vi "graph_data_acquisition_and_display.vi"(1 "input cluster":T2) -> (0 "output cluster":T1)   [LabVIEW 2015]
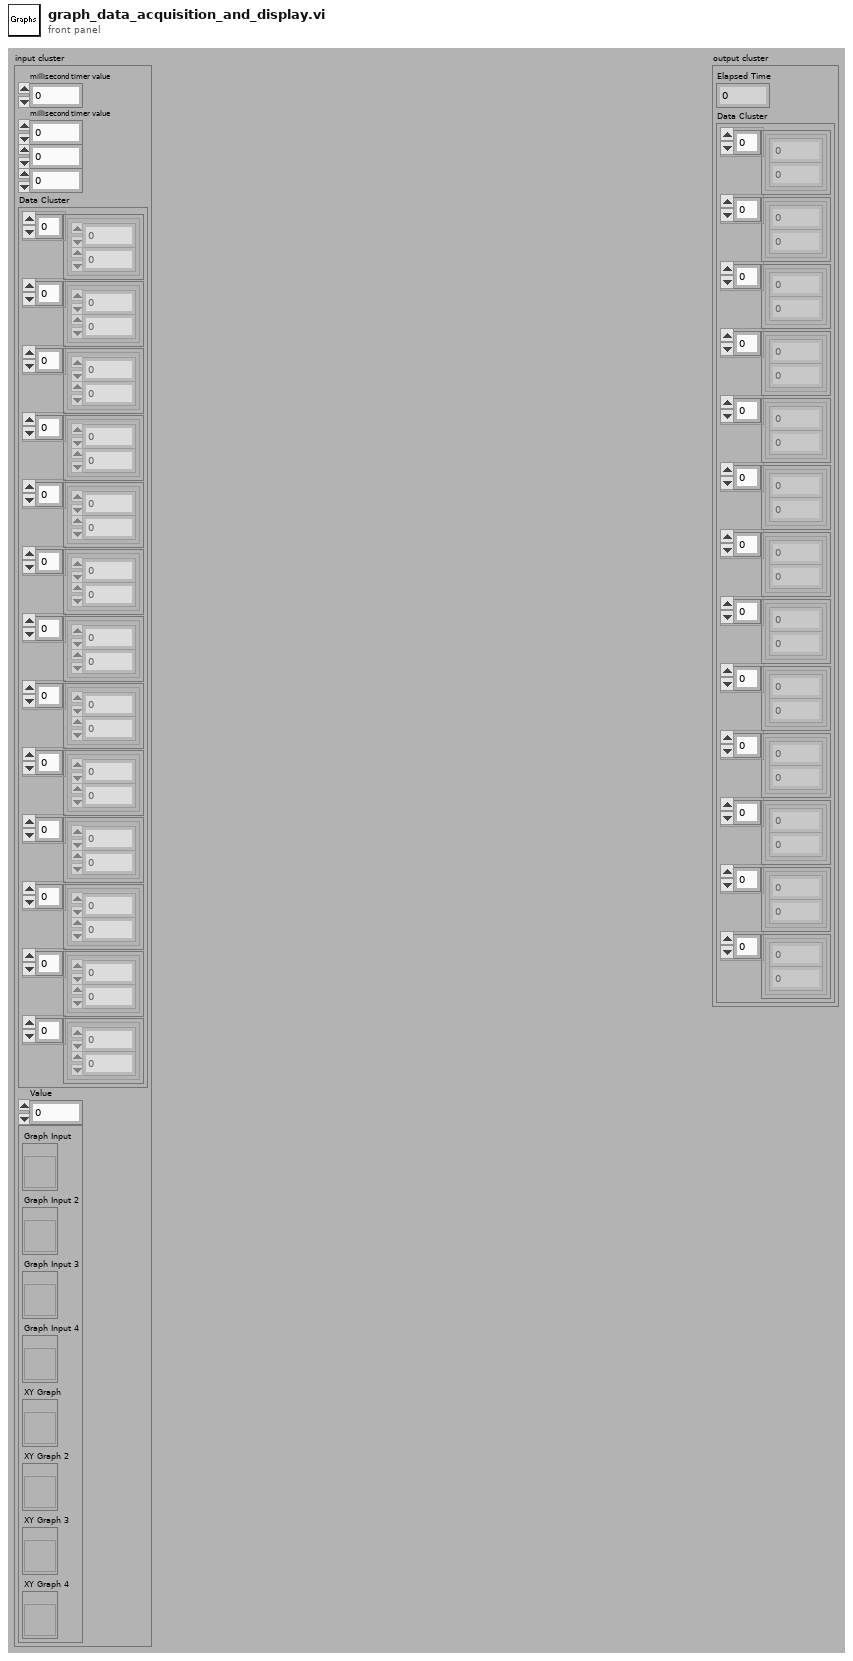
[diagram p1: front panel]
types:
  T1 = cluster{"Elapsed Time":i32, "Data Cluster":cluster{cluster{sgl, sgl}[], cluster{sgl, sgl}[], cluster{sgl, sgl}[], cluster{sgl, sgl}[], cluster{sgl, sgl}[], cluster{sgl, sgl}[], cluster{sgl, sgl}[], cluster{sgl, sgl}[], cluster{sgl, sgl}[], cluster{sgl, sgl}[], cluster{sgl, sgl}[], cluster{sgl, sgl}[], cluster{sgl, sgl}[]}}
  T2 = cluster{"millisecond timer value":u32, "millisecond timer value":u32, i32, sgl, "Data Cluster":cluster{cluster{sgl, sgl}[], cluster{sgl, sgl}[], cluster{sgl, sgl}[], cluster{sgl, sgl}[], cluster{sgl, sgl}[], cluster{sgl, sgl}[], cluster{sgl, sgl}[], cluster{sgl, sgl}[], cluster{sgl, sgl}[], cluster{sgl, sgl}[], cluster{sgl, sgl}[], cluster{sgl, sgl}[], cluster{sgl, sgl}[]}, "Value":i32, cluster{"Graph Input":refnum<vi>, "Graph Input 2":refnum<vi>, "Graph Input 3":refnum<vi>, "Graph Input 4":refnum<vi>, "XY Graph":refnum<vi>, "XY Graph 2":refnum<vi>, "XY Graph 3":refnum<vi>, "XY Graph 4":refnum<vi>}}
  T3 = cluster{cluster{sgl, sgl}[], cluster{sgl, sgl}[], cluster{sgl, sgl}[], cluster{sgl, sgl}[], cluster{sgl, sgl}[], cluster{sgl, sgl}[], cluster{sgl, sgl}[], cluster{sgl, sgl}[], cluster{sgl, sgl}[], cluster{sgl, sgl}[], cluster{sgl, sgl}[], cluster{sgl, sgl}[], cluster{sgl, sgl}[]}
  T4 = cluster{"Graph Input":refnum<vi>, "Graph Input 2":refnum<vi>, "Graph Input 3":refnum<vi>, "Graph Input 4":refnum<vi>, "XY Graph":refnum<vi>, "XY Graph 2":refnum<vi>, "XY Graph 3":refnum<vi>, "XY Graph 4":refnum<vi>}
  T5 = cluster{"Elapsed Time":i32, "output cluster":cluster{cluster{sgl, sgl}[], cluster{sgl, sgl}[], cluster{sgl, sgl}[], cluster{sgl, sgl}[], cluster{sgl, sgl}[], cluster{sgl, sgl}[], cluster{sgl, sgl}[], cluster{sgl, sgl}[], cluster{sgl, sgl}[], cluster{sgl, sgl}[], cluster{sgl, sgl}[], cluster{sgl, sgl}[], cluster{sgl, sgl}[]}}
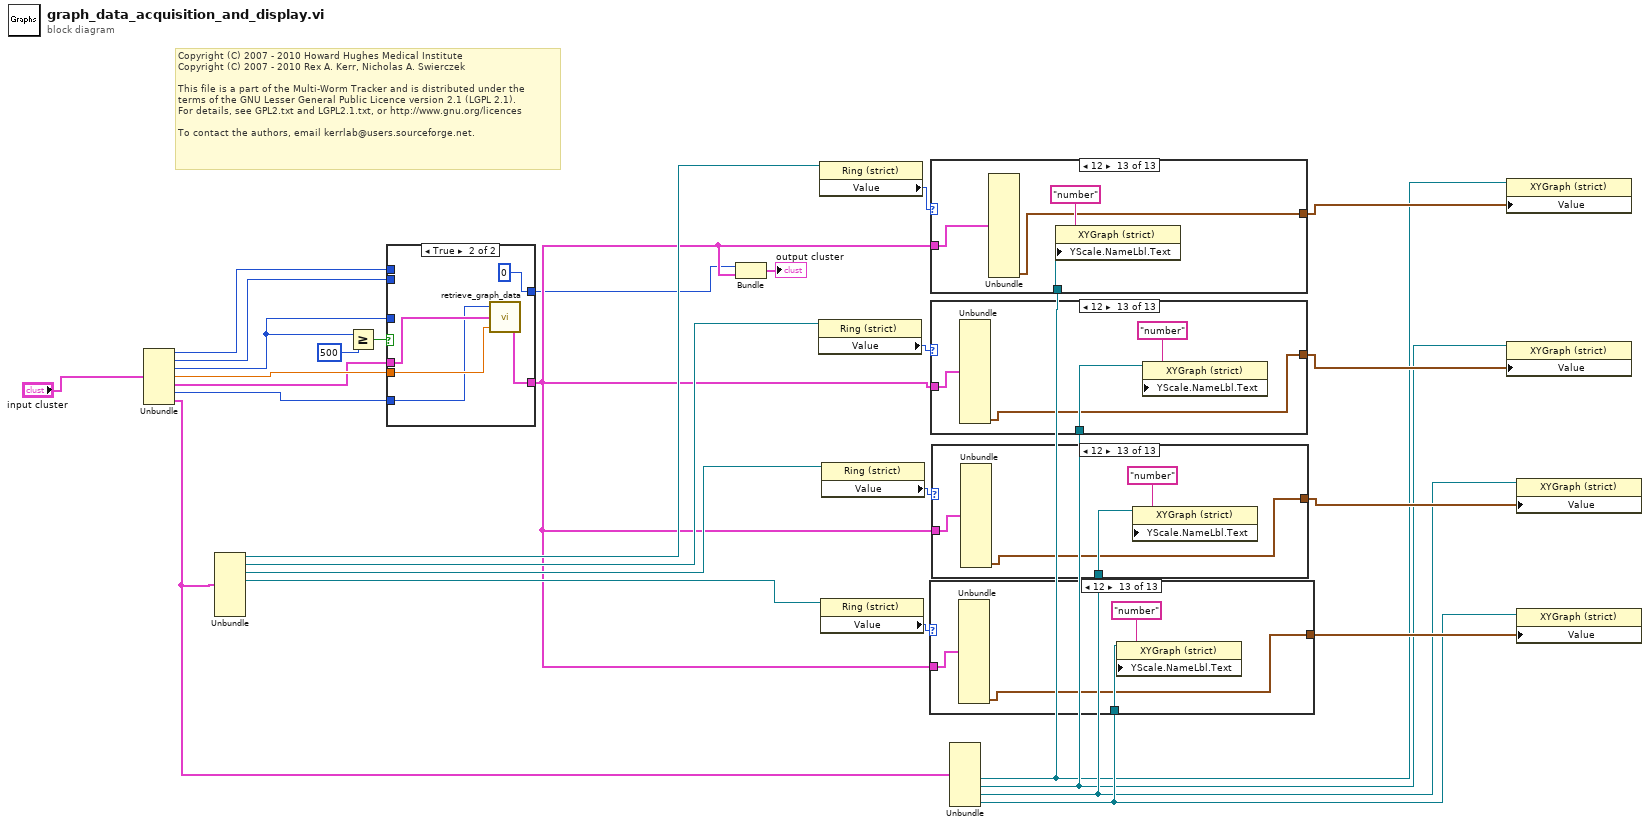
[diagram p0: block diagram]
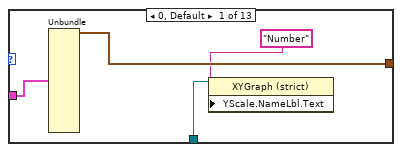
[diagram p2: hidden frame]
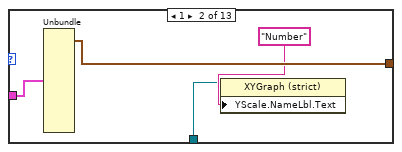
[diagram p3: hidden frame]
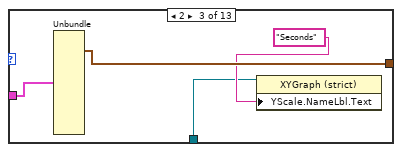
[diagram p4: hidden frame]
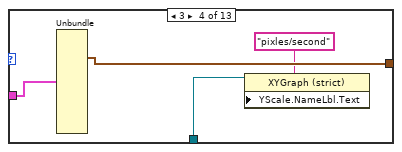
[diagram p5: hidden frame]
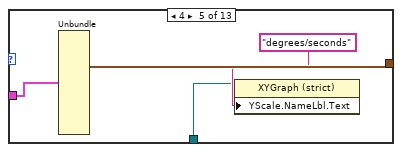
[diagram p6: hidden frame]
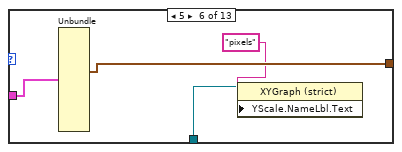
[diagram p7: hidden frame]
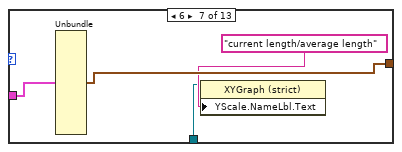
[diagram p8: hidden frame]
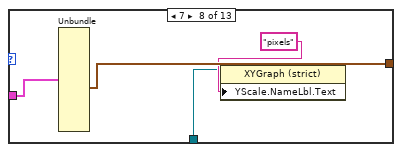
[diagram p9: hidden frame]
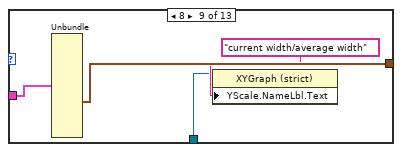
[diagram p10: hidden frame]
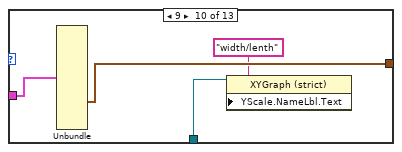
[diagram p11: hidden frame]
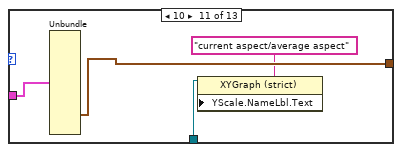
[diagram p12: hidden frame]
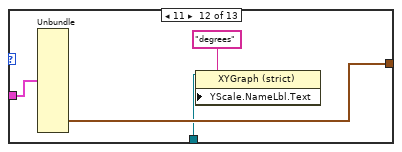
[diagram p13: hidden frame]
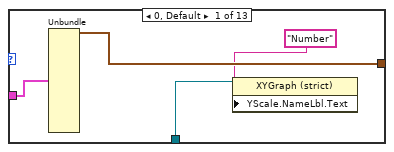
[diagram p14: hidden frame]
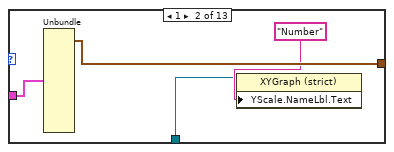
[diagram p15: hidden frame]
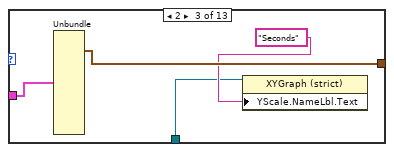
[diagram p16: hidden frame]
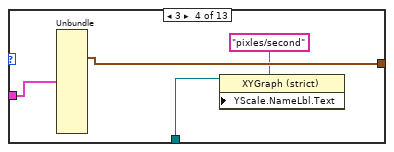
[diagram p17: hidden frame]
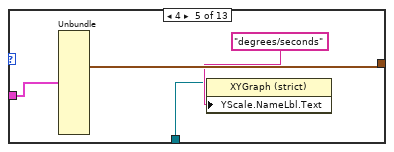
[diagram p18: hidden frame]
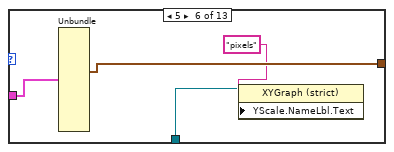
[diagram p19: hidden frame]
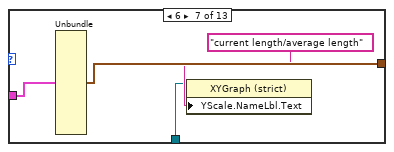
[diagram p20: hidden frame]
diagram:
  # "Copyright (C) 2007 - 2010 Howard Hughes Medical Institute\nCopyright (C) 2007 - 2010 Rex A. Kerr, Nicholas A. Swierczek\n \nThis file is a part of the Multi-Worm Tracker and is distributed under the\nterms of the GNU Lesser General Public Licence version 2.1 (LGPL 2.1).\nFor details, see GPL2.txt and LGPL2.1.txt, or http://www.gnu.org/licences\n \nTo contact the authors, email kerrlab@users.sourceforge.net."
  n1 = Unbundle("input cluster") -> ("millisecond timer value"=w14:u32, "millisecond timer value"=w13:u32, w12:i32, w11:sgl, "Data Cluster"=w10:T3, "Value"=w9:i32, w20:T4)
  n2 = Unbundle(w20) -> ("Graph Input"=w28:refnum<vi>, "Graph Input 2"=w26:refnum<vi>, "Graph Input 3"=w25:refnum<vi>, "Graph Input 4"=w24:refnum<vi>)  [unwired: 4 out]
  n3 = Greater Or Equal?(x=w12, y=500) -> (x >= y?=w5:bool)
  n4 = case shown="True" w5 {
    tunnel: [w30 0] -> w3
    tunnel: w12 -> [w31 _]
    tunnel: w14 -> [w33 _]
    tunnel: w13 -> [w32 _]
    tunnel: w11 -> [_ w38]
    tunnel: w10 -> [w34 w37]
    tunnel: [w34 w36] -> w4
    tunnel: w9 -> [_ w35]
    frame False {
      n5 = call "elapsed_time.vi"("Time since last update"=w31, "Initial Time"=w32, "Current Time"=w33) -> ("Elapsed Time"=w30:i32)
    }
    frame True {
      n6 = call "retrieve_graph_data.vi"("Time"=w38, "Data Cluster"=w37, "handle"=w35) -> ("output cluster"=w36:T3)
    }
  }
  n7 = Bundle("Elapsed Time"=w3, "output cluster"=w4) -> (→"output cluster":T5)  [unwired: 1 in]
  n8 = property class="Ring (strict)"(reference=w26) -> ("Value"=w23:u16)  [unwired: 1 in, 2 out]
  n9 = property class="Ring (strict)"(reference=w28) -> ("Value"=w27:u16)  [unwired: 1 in, 2 out]
  n10 = property class="Ring (strict)"(reference=w24) -> ("Value"=w21:u16)  [unwired: 1 in, 2 out]
  n11 = property class="Ring (strict)"(reference=w25) -> ("Value"=w22:u16)  [unwired: 1 in, 2 out]
  n12 = Unbundle(w20) -> ("XY Graph"=w6:refnum<vi>, "XY Graph 2"=w7:refnum<vi>, "XY Graph 3"=w8:refnum<vi>, "XY Graph 4"=w15:refnum<vi>)  [unwired: 4 out]
  n13 = case shown="12" w21 {
    tunnel: w4 -> [w43 w47 w51 w55 w59 w63 w67 w71 w75 w79 w83 w86 w90]
    tunnel: [w42 w46 w50 w54 w58 w62 w66 w70 w74 w78 w82 w85 w88] -> w16
    tunnel: w15 -> [w40 w44 w48 w52 w56 w60 w64 w68 w72 w76 w80 w84 w89]
    frame 0, Default {
      n14 = Unbundle(w43) -> (w42:cluster{sgl, sgl}[])  [unwired: 12 out]
      n15 = property on="Property Node" class="XYGraph (strict)"(reference=w40, "YScale.NameLbl.Text"="Number") -> ()  [unwired: 1 in, 2 out]
    }
    frame 1 {
      n16 = Unbundle(w47) -> (w46:cluster{sgl, sgl}[])  [unwired: 12 out]
      n17 = property on="Property Node" class="XYGraph (strict)"(reference=w44, "YScale.NameLbl.Text"="Number") -> ()  [unwired: 1 in, 2 out]
    }
    frame 2 {
      n18 = Unbundle(w51) -> (w50:cluster{sgl, sgl}[])  [unwired: 12 out]
      n19 = property on="Property Node" class="XYGraph (strict)"(reference=w48, "YScale.NameLbl.Text"="Seconds") -> ()  [unwired: 1 in, 2 out]
    }
    frame 3 {
      n20 = Unbundle(w55) -> (w54:cluster{sgl, sgl}[])  [unwired: 12 out]
      n21 = property on="Property Node" class="XYGraph (strict)"(reference=w52, "YScale.NameLbl.Text"="pixles/second") -> ()  [unwired: 1 in, 2 out]
    }
    frame 4 {
      n22 = Unbundle(w59) -> (w58:cluster{sgl, sgl}[])  [unwired: 12 out]
      n23 = property on="Property Node" class="XYGraph (strict)"(reference=w56, "YScale.NameLbl.Text"="degrees/seconds") -> ()  [unwired: 1 in, 2 out]
    }
    frame 5 {
      n24 = Unbundle(w63) -> (w62:cluster{sgl, sgl}[])  [unwired: 12 out]
      n25 = property on="Property Node" class="XYGraph (strict)"(reference=w60, "YScale.NameLbl.Text"="pixels") -> ()  [unwired: 1 in, 2 out]
    }
    frame 6 {
      n26 = Unbundle(w67) -> (w66:cluster{sgl, sgl}[])  [unwired: 12 out]
      n27 = property on="Property Node" class="XYGraph (strict)"(reference=w64, "YScale.NameLbl.Text"="current length/average length") -> ()  [unwired: 1 in, 2 out]
    }
    frame 7 {
      n28 = Unbundle(w71) -> (w70:cluster{sgl, sgl}[])  [unwired: 12 out]
      n29 = property on="Property Node" class="XYGraph (strict)"(reference=w68, "YScale.NameLbl.Text"="pixels") -> ()  [unwired: 1 in, 2 out]
    }
    frame 8 {
      n30 = Unbundle(w75) -> (w74:cluster{sgl, sgl}[])  [unwired: 12 out]
      n31 = property on="Property Node" class="XYGraph (strict)"(reference=w72, "YScale.NameLbl.Text"="current width/average width") -> ()  [unwired: 1 in, 2 out]
    }
    frame 9 {
      n32 = Unbundle(w79) -> (w78:cluster{sgl, sgl}[])  [unwired: 12 out]
      n33 = property on="Property Node" class="XYGraph (strict)"(reference=w76, "YScale.NameLbl.Text"="width/lenth") -> ()  [unwired: 1 in, 2 out]
    }
    frame 10 {
      n34 = Unbundle(w83) -> (w82:cluster{sgl, sgl}[])  [unwired: 12 out]
      n35 = property on="Property Node" class="XYGraph (strict)"(reference=w80, "YScale.NameLbl.Text"="current aspect/average aspect") -> ()  [unwired: 1 in, 2 out]
    }
    frame 11 {
      n36 = Unbundle(w86) -> (w85:cluster{sgl, sgl}[])  [unwired: 12 out]
      n37 = property on="Property Node" class="XYGraph (strict)"(reference=w84, "YScale.NameLbl.Text"="degrees") -> ()  [unwired: 1 in, 2 out]
    }
    frame 12 {
      n38 = Unbundle(w90) -> (w88:cluster{sgl, sgl}[])  [unwired: 12 out]
      n39 = property on="Property Node" class="XYGraph (strict)"(reference=w89, "YScale.NameLbl.Text"="number") -> ()  [unwired: 1 in, 2 out]
    }
  }
  n40 = case shown="12" w27 {
    tunnel: w4 -> [w95 w99 w103 w107 w111 w115 w119 w123 w127 w131 w135 w139 w143]
    tunnel: [w94 w98 w102 w106 w110 w114 w118 w122 w126 w130 w134 w138 w140] -> w19
    tunnel: w6 -> [w92 w96 w100 w104 w108 w112 w116 w120 w124 w128 w132 w136 w141]
    frame 0, Default {
      n41 = Unbundle(w95) -> (w94:cluster{sgl, sgl}[])  [unwired: 12 out]
      n42 = property on="Property Node" class="XYGraph (strict)"(reference=w92, "YScale.NameLbl.Text"="Number") -> ()  [unwired: 1 in, 2 out]
    }
    frame 1 {
      n43 = Unbundle(w99) -> (w98:cluster{sgl, sgl}[])  [unwired: 12 out]
      n44 = property on="Property Node" class="XYGraph (strict)"(reference=w96, "YScale.NameLbl.Text"="Number") -> ()  [unwired: 1 in, 2 out]
    }
    frame 2 {
      n45 = Unbundle(w103) -> (w102:cluster{sgl, sgl}[])  [unwired: 12 out]
      n46 = property on="Property Node" class="XYGraph (strict)"(reference=w100, "YScale.NameLbl.Text"="Seconds") -> ()  [unwired: 1 in, 2 out]
    }
    frame 3 {
      n47 = Unbundle(w107) -> (w106:cluster{sgl, sgl}[])  [unwired: 12 out]
      n48 = property on="Property Node" class="XYGraph (strict)"(reference=w104, "YScale.NameLbl.Text"="pixles/second") -> ()  [unwired: 1 in, 2 out]
    }
    frame 4 {
      n49 = Unbundle(w111) -> (w110:cluster{sgl, sgl}[])  [unwired: 12 out]
      n50 = property on="Property Node" class="XYGraph (strict)"(reference=w108, "YScale.NameLbl.Text"="degrees/seconds") -> ()  [unwired: 1 in, 2 out]
    }
    frame 5 {
      n51 = Unbundle(w115) -> (w114:cluster{sgl, sgl}[])  [unwired: 12 out]
      n52 = property on="Property Node" class="XYGraph (strict)"(reference=w112, "YScale.NameLbl.Text"="pixels") -> ()  [unwired: 1 in, 2 out]
    }
    frame 6 {
      n53 = Unbundle(w119) -> (w118:cluster{sgl, sgl}[])  [unwired: 12 out]
      n54 = property on="Property Node" class="XYGraph (strict)"(reference=w116, "YScale.NameLbl.Text"="current length/average length") -> ()  [unwired: 1 in, 2 out]
    }
    frame 7 {
      n55 = Unbundle(w123) -> (w122:cluster{sgl, sgl}[])  [unwired: 12 out]
      n56 = property on="Property Node" class="XYGraph (strict)"(reference=w120, "YScale.NameLbl.Text"="pixels") -> ()  [unwired: 1 in, 2 out]
    }
    frame 8 {
      n57 = Unbundle(w127) -> (w126:cluster{sgl, sgl}[])  [unwired: 12 out]
      n58 = property on="Property Node" class="XYGraph (strict)"(reference=w124, "YScale.NameLbl.Text"="current width/average width") -> ()  [unwired: 1 in, 2 out]
    }
    frame 9 {
      n59 = Unbundle(w131) -> (w130:cluster{sgl, sgl}[])  [unwired: 12 out]
      n60 = property on="Property Node" class="XYGraph (strict)"(reference=w128, "YScale.NameLbl.Text"="width/lenth") -> ()  [unwired: 1 in, 2 out]
    }
    frame 10 {
      n61 = Unbundle(w135) -> (w134:cluster{sgl, sgl}[])  [unwired: 12 out]
      n62 = property on="Property Node" class="XYGraph (strict)"(reference=w132, "YScale.NameLbl.Text"="current aspect/average aspect") -> ()  [unwired: 1 in, 2 out]
    }
    frame 11 {
      n63 = Unbundle(w139) -> (w138:cluster{sgl, sgl}[])  [unwired: 12 out]
      n64 = property on="Property Node" class="XYGraph (strict)"(reference=w136, "YScale.NameLbl.Text"="degrees") -> ()  [unwired: 1 in, 2 out]
    }
    frame 12 {
      n65 = Unbundle(w143) -> (w140:cluster{sgl, sgl}[])  [unwired: 12 out]
      n66 = property on="Property Node" class="XYGraph (strict)"(reference=w141, "YScale.NameLbl.Text"="number") -> ()  [unwired: 1 in, 2 out]
    }
  }
  n67 = case shown="12" w23 {
    tunnel: w4 -> [w147 w151 w155 w159 w163 w167 w171 w175 w179 w183 w187 w190 w194]
    tunnel: [w146 w150 w154 w158 w162 w166 w170 w174 w178 w182 w186 w189 w192] -> w18
    tunnel: w7 -> [w144 w148 w152 w156 w160 w164 w168 w172 w176 w180 w184 w188 w193]
    frame 0, Default {
      n68 = Unbundle(w147) -> (w146:cluster{sgl, sgl}[])  [unwired: 12 out]
      n69 = property on="Property Node" class="XYGraph (strict)"(reference=w144, "YScale.NameLbl.Text"="Number") -> ()  [unwired: 1 in, 2 out]
    }
    frame 1 {
      n70 = Unbundle(w151) -> (w150:cluster{sgl, sgl}[])  [unwired: 12 out]
      n71 = property on="Property Node" class="XYGraph (strict)"(reference=w148, "YScale.NameLbl.Text"="Number") -> ()  [unwired: 1 in, 2 out]
    }
    frame 2 {
      n72 = Unbundle(w155) -> (w154:cluster{sgl, sgl}[])  [unwired: 12 out]
      n73 = property on="Property Node" class="XYGraph (strict)"(reference=w152, "YScale.NameLbl.Text"="Seconds") -> ()  [unwired: 1 in, 2 out]
    }
    frame 3 {
      n74 = Unbundle(w159) -> (w158:cluster{sgl, sgl}[])  [unwired: 12 out]
      n75 = property on="Property Node" class="XYGraph (strict)"(reference=w156, "YScale.NameLbl.Text"="pixles/second") -> ()  [unwired: 1 in, 2 out]
    }
    frame 4 {
      n76 = Unbundle(w163) -> (w162:cluster{sgl, sgl}[])  [unwired: 12 out]
      n77 = property on="Property Node" class="XYGraph (strict)"(reference=w160, "YScale.NameLbl.Text"="degrees/seconds") -> ()  [unwired: 1 in, 2 out]
    }
    frame 5 {
      n78 = Unbundle(w167) -> (w166:cluster{sgl, sgl}[])  [unwired: 12 out]
      n79 = property on="Property Node" class="XYGraph (strict)"(reference=w164, "YScale.NameLbl.Text"="pixels") -> ()  [unwired: 1 in, 2 out]
    }
    frame 6 {
      n80 = Unbundle(w171) -> (w170:cluster{sgl, sgl}[])  [unwired: 12 out]
      n81 = property on="Property Node" class="XYGraph (strict)"(reference=w168, "YScale.NameLbl.Text"="current length/average length") -> ()  [unwired: 1 in, 2 out]
    }
    frame 7 {
      n82 = Unbundle(w175) -> (w174:cluster{sgl, sgl}[])  [unwired: 12 out]
      n83 = property on="Property Node" class="XYGraph (strict)"(reference=w172, "YScale.NameLbl.Text"="pixels") -> ()  [unwired: 1 in, 2 out]
    }
    frame 8 {
      n84 = Unbundle(w179) -> (w178:cluster{sgl, sgl}[])  [unwired: 12 out]
      n85 = property on="Property Node" class="XYGraph (strict)"(reference=w176, "YScale.NameLbl.Text"="current width/average width") -> ()  [unwired: 1 in, 2 out]
    }
    frame 9 {
      n86 = Unbundle(w183) -> (w182:cluster{sgl, sgl}[])  [unwired: 12 out]
      n87 = property on="Property Node" class="XYGraph (strict)"(reference=w180, "YScale.NameLbl.Text"="width/lenth") -> ()  [unwired: 1 in, 2 out]
    }
    frame 10 {
      n88 = Unbundle(w187) -> (w186:cluster{sgl, sgl}[])  [unwired: 12 out]
      n89 = property on="Property Node" class="XYGraph (strict)"(reference=w184, "YScale.NameLbl.Text"="current aspect/average aspect") -> ()  [unwired: 1 in, 2 out]
    }
    frame 11 {
      n90 = Unbundle(w190) -> (w189:cluster{sgl, sgl}[])  [unwired: 12 out]
      n91 = property on="Property Node" class="XYGraph (strict)"(reference=w188, "YScale.NameLbl.Text"="degrees") -> ()  [unwired: 1 in, 2 out]
    }
    frame 12 {
      n92 = Unbundle(w194) -> (w192:cluster{sgl, sgl}[])  [unwired: 12 out]
      n93 = property on="Property Node" class="XYGraph (strict)"(reference=w193, "YScale.NameLbl.Text"="number") -> ()  [unwired: 1 in, 2 out]
    }
  }
  n94 = case shown="12" w22 {
    tunnel: w4 -> [w199 w203 w207 w211 w215 w219 w223 w227 w231 w235 w239 w242 w246]
    tunnel: [w198 w202 w206 w210 w214 w218 w222 w226 w230 w234 w238 w241 w244] -> w17
    tunnel: w8 -> [w196 w200 w204 w208 w212 w216 w220 w224 w228 w232 w236 w240 w245]
    frame 0, Default {
      n95 = Unbundle(w199) -> (w198:cluster{sgl, sgl}[])  [unwired: 12 out]
      n96 = property on="Property Node" class="XYGraph (strict)"(reference=w196, "YScale.NameLbl.Text"="Number") -> ()  [unwired: 1 in, 2 out]
    }
    frame 1 {
      n97 = Unbundle(w203) -> (w202:cluster{sgl, sgl}[])  [unwired: 12 out]
      n98 = property on="Property Node" class="XYGraph (strict)"(reference=w200, "YScale.NameLbl.Text"="Number") -> ()  [unwired: 1 in, 2 out]
    }
    frame 2 {
      n99 = Unbundle(w207) -> (w206:cluster{sgl, sgl}[])  [unwired: 12 out]
      n100 = property on="Property Node" class="XYGraph (strict)"(reference=w204, "YScale.NameLbl.Text"="Seconds") -> ()  [unwired: 1 in, 2 out]
    }
    frame 3 {
      n101 = Unbundle(w211) -> (w210:cluster{sgl, sgl}[])  [unwired: 12 out]
      n102 = property on="Property Node" class="XYGraph (strict)"(reference=w208, "YScale.NameLbl.Text"="pixles/second") -> ()  [unwired: 1 in, 2 out]
    }
    frame 4 {
      n103 = Unbundle(w215) -> (w214:cluster{sgl, sgl}[])  [unwired: 12 out]
      n104 = property on="Property Node" class="XYGraph (strict)"(reference=w212, "YScale.NameLbl.Text"="degrees/seconds") -> ()  [unwired: 1 in, 2 out]
    }
    frame 5 {
      n105 = Unbundle(w219) -> (w218:cluster{sgl, sgl}[])  [unwired: 12 out]
      n106 = property on="Property Node" class="XYGraph (strict)"(reference=w216, "YScale.NameLbl.Text"="pixels") -> ()  [unwired: 1 in, 2 out]
    }
    frame 6 {
      n107 = Unbundle(w223) -> (w222:cluster{sgl, sgl}[])  [unwired: 12 out]
      n108 = property on="Property Node" class="XYGraph (strict)"(reference=w220, "YScale.NameLbl.Text"="current length/average length") -> ()  [unwired: 1 in, 2 out]
    }
    frame 7 {
      n109 = Unbundle(w227) -> (w226:cluster{sgl, sgl}[])  [unwired: 12 out]
      n110 = property on="Property Node" class="XYGraph (strict)"(reference=w224, "YScale.NameLbl.Text"="pixels") -> ()  [unwired: 1 in, 2 out]
    }
    frame 8 {
      n111 = Unbundle(w231) -> (w230:cluster{sgl, sgl}[])  [unwired: 12 out]
      n112 = property on="Property Node" class="XYGraph (strict)"(reference=w228, "YScale.NameLbl.Text"="current width/average width") -> ()  [unwired: 1 in, 2 out]
    }
    frame 9 {
      n113 = Unbundle(w235) -> (w234:cluster{sgl, sgl}[])  [unwired: 12 out]
      n114 = property on="Property Node" class="XYGraph (strict)"(reference=w232, "YScale.NameLbl.Text"="width/lenth") -> ()  [unwired: 1 in, 2 out]
    }
    frame 10 {
      n115 = Unbundle(w239) -> (w238:cluster{sgl, sgl}[])  [unwired: 12 out]
      n116 = property on="Property Node" class="XYGraph (strict)"(reference=w236, "YScale.NameLbl.Text"="current aspect/average aspect") -> ()  [unwired: 1 in, 2 out]
    }
    frame 11 {
      n117 = Unbundle(w242) -> (w241:cluster{sgl, sgl}[])  [unwired: 12 out]
      n118 = property on="Property Node" class="XYGraph (strict)"(reference=w240, "YScale.NameLbl.Text"="degrees") -> ()  [unwired: 1 in, 2 out]
    }
    frame 12 {
      n119 = Unbundle(w246) -> (w244:cluster{sgl, sgl}[])  [unwired: 12 out]
      n120 = property on="Property Node" class="XYGraph (strict)"(reference=w245, "YScale.NameLbl.Text"="number") -> ()  [unwired: 1 in, 2 out]
    }
  }
  n121 = property class="XYGraph (strict)"(reference=w6, "Value"=w19) -> ()  [unwired: 1 in, 2 out]
  n122 = property class="XYGraph (strict)"(reference=w7, "Value"=w18) -> ()  [unwired: 1 in, 2 out]
  n123 = property class="XYGraph (strict)"(reference=w8, "Value"=w17) -> ()  [unwired: 1 in, 2 out]
  n124 = property class="XYGraph (strict)"(reference=w15, "Value"=w16) -> ()  [unwired: 1 in, 2 out]
